vi "smoothing_matrix.vi"(1 "Smoothing Parameter (Gaussian S.D. in pixels)":dbl, 2 "Size":i32) -> (0 "Smoothing Matrix":dbl[][](graph))   [LabVIEW 2010]
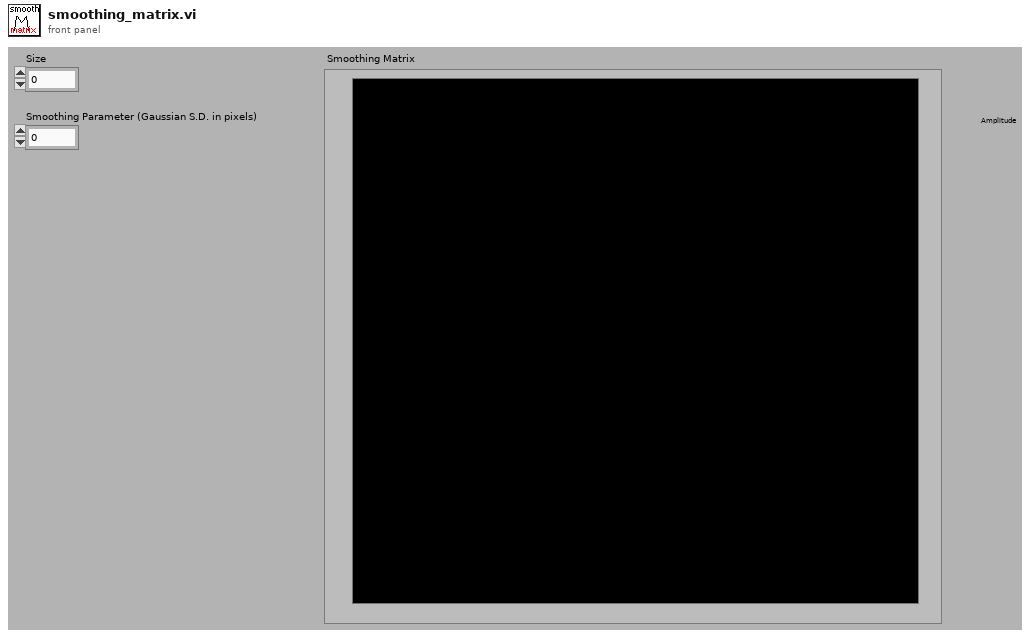
[diagram p1: front panel]
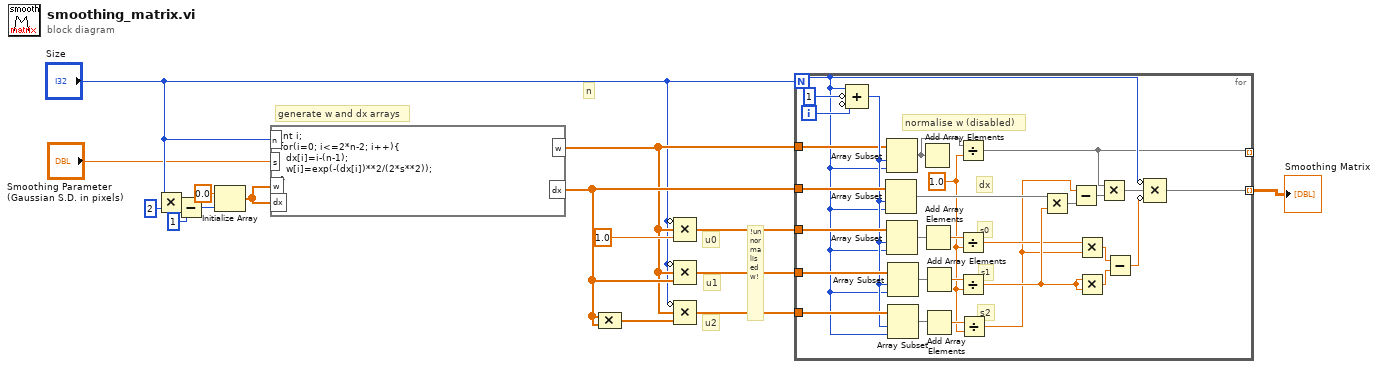
[diagram p0: block diagram]
diagram:
  # "!unnormalised w!"
  # "u2"
  # "u1"
  # "u0"
  # "n"
  # "generate w and dx arrays"
  n1 = Multiply(x="Size", y=2) -> (x*y=w5:i32)
  n2 = Subtract(x=w5, y=1) -> (x-y=w4:i32)
  n3 = Initialize Array(0.0 ("element"), w4) -> (w3:dbl[])
  n4 = formula code="int i;\nfor(i=0; i<=2*n-2; i++){\n  dx[i]=i-(n-1);\n  w[i]=exp(-(dx[i])**2/(2*s**2));\n}"("s"="Smoothing Parameter (Gaussian S.D. in pixels)", "n"="Size", "w"=w3, "dx"=w3) -> ("w"=w10:dbl[], "dx"=w13:dbl[])
  n5 = Compound Arithmetic op=MULTIPLY(w13, w13) -> (w12:dbl[])
  n6 = Compound Arithmetic op=MULTIPLY(invert "Size", w10, 1.0) -> (w11:dbl[])
  n7 = Compound Arithmetic op=MULTIPLY(invert "Size", w10, w13) -> (w15:dbl[])
  n8 = Compound Arithmetic op=MULTIPLY(invert "Size", w10, w12) -> (w16:dbl[])
  n9 = for {
    N: "Size" -> [w20]
    tunnel: w16 -> [w40]
    tunnel: w15 -> [w41]
    tunnel: w11 -> [w42]
    tunnel: w13 -> [w45]
    tunnel: w10 -> [w35]
    tunnel: [w21] -> w8 mode=indexing
    tunnel: [w19] -> _ mode=indexing
    i -> [w44]
    w17 = 1.0
    # "dx"
    # "s2"
    # "s0"
    # "s1"
    # "normalise w (disabled)"
    n10 = Compound Arithmetic op=ADD(w20, invert 1 ("value"), invert w44) -> (w39:i32)
    n11 = Array Subset(array=w45, index=w39, length=w20) -> (w30:dbl[])
    n12 = Array Subset(array=w35, index=w39, length=w20) -> (w18:dbl[])
    n13 = Array Subset(array=w42, index=w39, length=w20) -> (w38:dbl[])
    n14 = Array Subset(array=w41, index=w39, length=w20) -> (w37:dbl[])
    n15 = Array Subset(array=w40, index=w39, length=w20) -> (w36:dbl[])
    n16 = Add Array Elements(numeric array=w18) -> ()  [unwired: 1 out]
    n17 = Add Array Elements(numeric array=w38) -> (sum=w31:dbl)
    n18 = Add Array Elements(numeric array=w37) -> (sum=w32:dbl)
    n19 = Add Array Elements(numeric array=w36) -> (sum=w33:dbl)
    n20 = Divide(x=w18, y=w17) -> (x/y=w19:dbl[])
    n21 = Divide(x=w31, y=w17) -> (x/y=w26:dbl)
    n22 = Divide(x=w32, y=w17) -> (x/y=w27:dbl)
    n23 = Divide(x=w33, y=w17) -> (x/y=w25:dbl)
    n24 = Multiply(x=w30, y=w27) -> (x*y=w34:dbl[])
    n25 = Subtract(x=w25, y=w34) -> (x-y=w29:dbl[])
    n26 = Multiply(x=w26, y=w25) -> (x*y=w23:dbl)
    n27 = Multiply(x=w27, y=w27) -> (x*y=w24:dbl)
    n28 = Multiply(x=w19, y=w29) -> (x*y=w28:dbl[])
    n29 = Subtract(x=w23, y=w24) -> (x-y=w22:dbl)
    n30 = Compound Arithmetic op=MULTIPLY(invert w20, w28, invert w22) -> (w21:dbl[])
  }
  "Smoothing Matrix" <- w8
